vi "CFG_PumpParams.vi"(11 "all rows":string[][](array[string])) -> (3 "Pump Params":T1 {"Sim Fill Rate" format="%.3f"; "Laser Offset" format="%.3f"; "Laser Slope" format="%.3f"; "RNG_STOP" format="%#_13g"; "RNG_CREEP" format="%#_13g"; "RNG_SLOW" format="%#_13g"})   [LabVIEW 2024]
uses:
  DEF_PumpParams.ctl
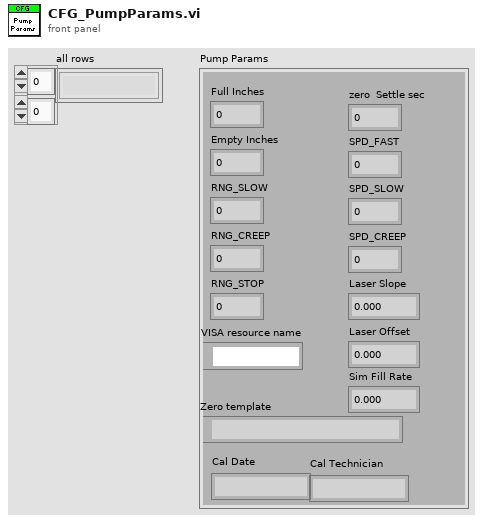
[diagram p1: front panel]
types:
  T1 = typedef "DEF_PumpParams.ctl" = cluster{"Empty Inches":dbl, "Full Inches":dbl, "RNG_SLOW":dbl, "RNG_CREEP":dbl, "RNG_STOP ":dbl, "VISA resource name":refnum<visa-resource-name>, "SPD_SLOW":i32, "SPD_CREEP":i32, "SPD_FAST":i32, "Zero template":path, "zero  Settle sec":i32, "Laser Slope":sgl, "Laser Offset":sgl, "Sim Fill Rate":sgl, "Cal Date":string, "Cal Technician":string}
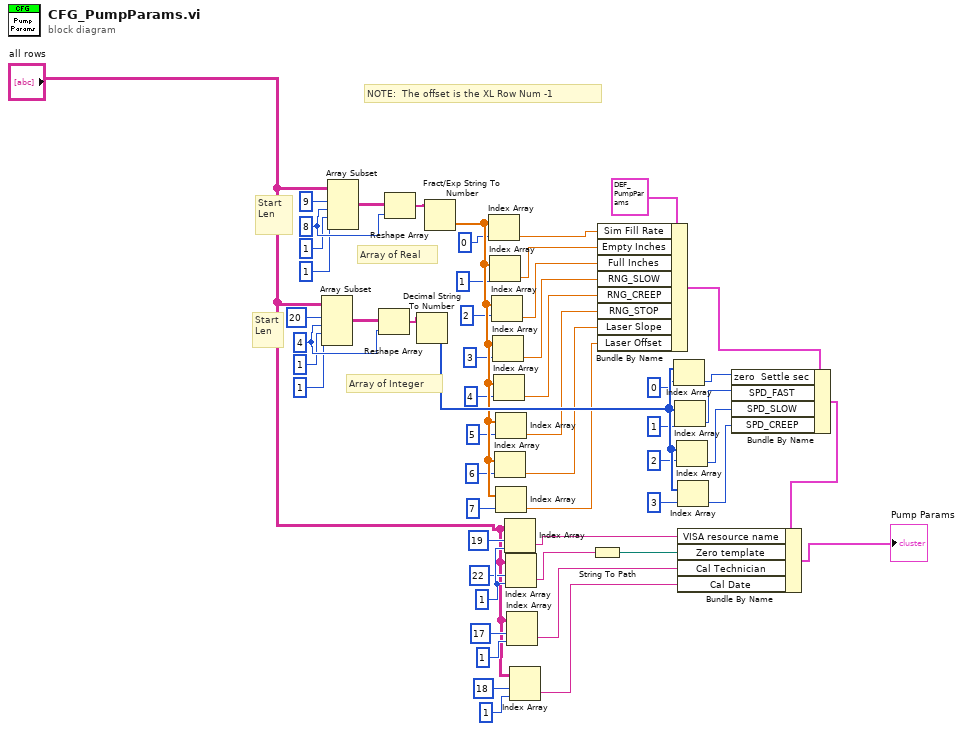
[diagram p0: block diagram]
diagram:
  w51 = 1 ("disabled index (col)")
  w35 = 4 ("index")
  w36 = 8 ("index")
  # "NOTE:  The offset is the XL Row Num -1"
  # "Array of Integer"
  # "Array of Real"
  # "Start\nLen"
  # "Start\nLen"
  n1 = Array Subset(array="all rows", index (row)=20 ("index"), length (row)=w35, index (col)=1 ("index"), length (col)=1 ("index")) -> (w34:string[][])
  n2 = Array Subset(array="all rows", index (row)=9 ("index"), length (row)=w36, index (col)=1 ("index"), length (col)=1 ("index")) -> (w19:string[][])
  n3 = Reshape Array(w34, w35) -> (w41:string[])
  n4 = Reshape Array(w19, w36) -> (w20:string[])
  n5 = Decimal String To Number(string=w41) -> (number=w42:i32[])  [unwired: 2 in, 1 out]
  n6 = Fract/Exp String To Number(string=w20) -> (number=w29:dbl[])  [unwired: 3 in, 1 out]
  n7 = Index Array(array=w29, index=0) -> (element=w18:dbl)
  n8 = Index Array(array=w29, index=1) -> (element=w21:dbl)
  n9 = Index Array(array=w29, index=2) -> (element=w22:dbl)
  n10 = Index Array(array=w29, index=3) -> (element=w23:dbl)
  n11 = Index Array(array=w29, index=4) -> (element=w24:dbl)
  n12 = Index Array(array=w29, index=6) -> (element=w27:dbl)
  n13 = Index Array(array=w29, index=5) -> (element=w25:dbl)
  n14 = Index Array(array=w29, index=7) -> (element=w30:dbl)
  n15 = Index Array(array="all rows", index (row)=19 ("index"), index (col)=w51) -> (element=w52:string)
  n16 = Index Array(array="all rows", index (row)=22 ("index"), index (col)=w51) -> (element=w53:string)
  n17 = Index Array(array="all rows", index (row)=17 ("index"), index (col)=1 ("disabled index (col)")) -> (element=w2:string)
  n18 = Index Array(array="all rows", index (row)=18 ("index"), index (col)=1 ("disabled index (col)")) -> (element=w1:string)
  n19 = String To Path(string=w53) -> (path=w54:path)
  n20 = Bundle By Name(cluster=T1 {"Empty Inches"=0.0, "Full Inches"=0.0, "RNG_SLOW"=0.5, "RNG_CREEP"=0.007, "RNG_STOP "=0.002, "VISA resource name"="COM4", "SPD_SLOW"=0, "SPD_CREEP"=0, "SPD_FAST"=0, "Zero template"=path "C:/AllenProjects/PWC-OLS/$Calibrtation/CAL_Level_RnR_241105.xlsx", "zero  Settle sec"=0, "Laser Slope"=0.0, "Laser Offset"=0.0, "Sim Fill Rate"=0.0, "Cal Date"="", "Cal Technician"=""} ("Pump Params"), "Sim Fill Rate"=w18, "Empty Inches"=w21, "Full Inches"=w22, "RNG_SLOW"=w23, "RNG_CREEP"=w24, "RNG_STOP"=w25, "Laser Slope"=w27, "Laser Offset"=w30) -> (w43:T1)
  n21 = Index Array(array=w42, index=0) -> (element=w44:i32)
  n22 = Index Array(array=w42, index=1) -> (element=w45:i32)
  n23 = Index Array(array=w42, index=2) -> (element=w46:i32)
  n24 = Index Array(array=w42, index=3) -> (element=w47:i32)
  n25 = Bundle By Name(cluster=w43, "zero  Settle sec"=w44, "SPD_FAST"=w45, "SPD_SLOW"=w46, "SPD_CREEP"=w47) -> (w50:T1)
  n26 = Bundle By Name(cluster=w50, "VISA resource name"=w52, "Zero template"=w54, "Cal Technician"=w2, "Cal Date"=w1) -> (→"Pump Params":T1)
